vi "Recursive Owned VIs List.vi"(11 "Parent[]":refnum<vi>[](array[refnum])) -> (3 "Children[]":refnum<vi>[](array[refnum]))   [LabVIEW 2015, in "TLB` Springboard.lvlib"]
uses:
  TLB` Springboard.lvlib
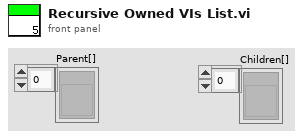
[diagram p1: front panel]
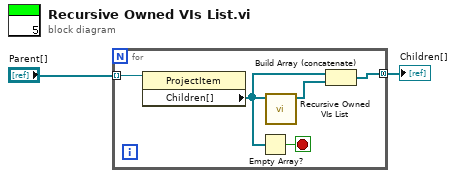
[diagram p0: block diagram]
diagram:
  n1 = for {
    tunnel: "Parent[]" -> [w7] mode=indexing
    tunnel: [w4] -> w1 mode=concatenating
    stop <- w6 stop-if-true
    n2 = property class="ProjectItem"(reference=w7) -> ("Children[]"=w5:refnum<vi>[])  [unwired: 1 in, 2 out]
    n3 = Empty Array?(array=w5) -> (empty?=w6:bool)
    n4 = call "Recursive Owned VIs List.vi"("Parent[]"=w5) -> ("Children[]"=w3:refnum<vi>[])  [unwired: 10 in]
    n5 = Build Array (concatenate)(w5, w3) -> (w4:refnum<vi>[])
  }
  "Children[]" <- w1
